vi "Movimiento_1Eje(SubVi).vi"(1 "Velocidad":dbl, 2 "Posición":dbl, 3 "Motion Resource 1":refnum<k21>="Eje X") -> (0 "Done":bool)   [LabVIEW 2017]
uses:
  <vilib>/Motion/Express/_s/nimc.fb.straightLineMove.startStraightLineMove.axis.modeAbsolute.0.vi
  <vilib>/Motion/BlockNode/FB.NIMotion.xnode
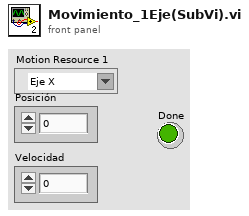
[diagram p1: front panel]
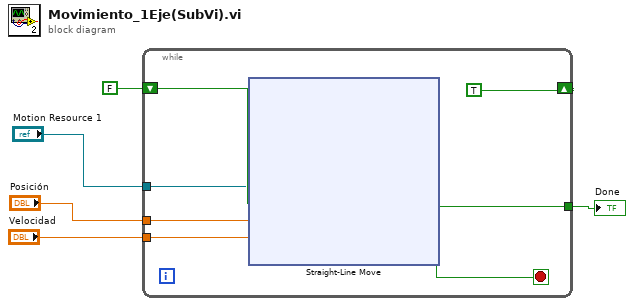
[diagram p0: block diagram]
diagram:
  n1 = while {
    shift-right: [TRUE] -> _
    shift-left: FALSE -> [w10]
    tunnel: [w9] -> w4
    tunnel: "Velocidad" -> [w8]
    tunnel: "Posición" -> [w7]
    tunnel: "Motion Resource 1" -> [w6]
    stop <- w9 stop-if-true
    n2 = xnode "Straight-Line Move"("resource"=w6, "execute"=w10, "position"=w7, "velocity"=w8) -> ("done"=w9:bool)  [unwired: 2 in, 2 out]
  }
  "Done" <- w4
